vi "Load Patterns from Library.vi"(8 "error in (no error)":errorcluster, 11 "MultiPattern Matcher in":refnum<class "MultiPattern Matcher.lvclass">) -> (0 "error out":errorcluster, 3 "MultiPattern Matcher out":refnum<class "MultiPattern Matcher.lvclass">)   [LabVIEW 2013, in "MultiPattern Matcher.lvclass"]
uses:
  MultiPattern Matcher.lvclass
  <vilib>/vision/Image Controls.llb/IMAQ Image.ctl
  MultiPattern Matcher.lvclass/MultiPattern Matcher.ctl
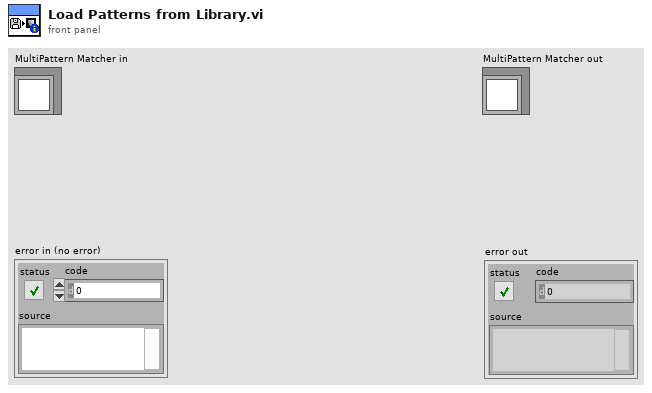
[diagram p1: front panel]
types:
  T1 = typedef "IMAQ Image.ctl" = refnum<image>
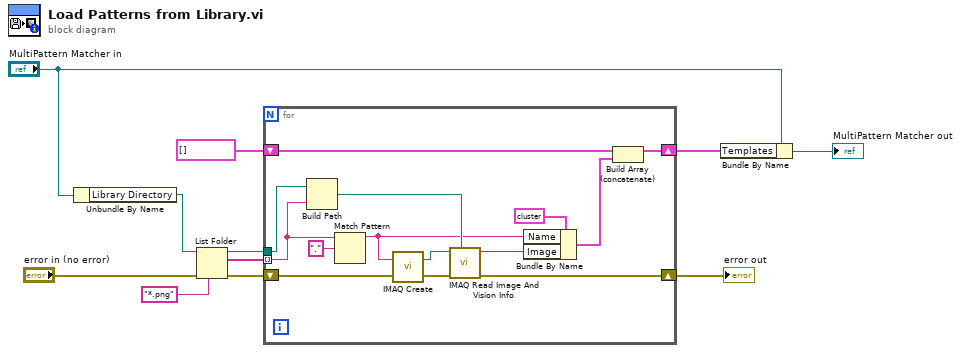
[diagram p0: block diagram]
diagram:
  n1 = Unbundle By Name("MultiPattern Matcher in") -> ("Library Directory"=w9:path)
  n2 = List Folder(path=w9, pattern="*.png", error in="error in (no error)") -> (path out=w7:path, filenames=w6:string[], error out=w8:errorcluster)  [unwired: 1 in, 1 out]
  n3 = for {
    tunnel: w7 -> [w25]
    tunnel: w6 -> [w19] mode=indexing
    shift-right: [w13] -> w2
    shift-left: w8 -> [w23]
    shift-right: [w17] -> w3
    shift-left: cluster{"Image":T1, "Name":string}[] [] ("Templates") -> [w18]
    n4 = Build Path(base path=w25, name or relative path=w19) -> (appended path=w24:path)
    n5 = Match Pattern(string=w19, regular expression=".") -> (before substring=w14:string)  [unwired: 1 in, 3 out]
    n6 = call "IMAQ Create"("Image Name"=w14, "error in (no error)"=w23) -> ("New Image"=w21:T1, "error out"=w22:errorcluster)  [unwired: 3 in]
    n7 = call "IMAQ Read Image And Vision Info"("File Path"=w24, "error in (no error)"=w22, "Image"=w21) -> ("error out"=w13:errorcluster, "Image Out"=w15:T1)  [unwired: 6 in, 1 out]
    n8 = Bundle By Name(cluster=cluster{"Image":T1, "Name":string} {"Image"=refnum, "Name"=""} ("Cluster"), "Name"=w14, "Image"=w15) -> (w12:cluster{"Image":T1, "Name":string})
    n9 = Build Array (concatenate)(w18, w12) -> (w17:cluster{"Image":T1, "Name":string}[])
  }
  "error out" <- w2
  n10 = Bundle By Name(cluster="MultiPattern Matcher in", "Templates"=w3) -> (→"MultiPattern Matcher out":refnum<class "MultiPattern Matcher.lvclass">)
